vi "PH_PSDBWriter.get PSDB Instance ID.vi"(0 "i ref in":refnum<vi>, 2 "Subsystem":T2 caption="PHELIX Subsysteme" items=["Miscellaneous", "fs-Frontend", "ns-Frontend", "PreAmp", "MainAmp", "MAS", "COS", "Beamline", "Experiment Laserbay", "Experiment Laserlabor", "Experiment Z6", "Timing", "Pulsed Power"], 5 "error in":errorcluster) -> (14 "i ref out":refnum<vi>, 16 "Metadata.Data Status":T1 items=["no info", "no Data collection", "no problem", "Error getting the ID", "Error writing Data", "Error getting the subsystem", "Error getting the Shot ID", "Error getting the Shot Types", "Error getting the Experiments", "Error verifying wanted Shottype", "Error verifying wanted Experiment"], 17 "instance_id":i32, 18 "PSDB Error Code":i32, 19 "error out":errorcluster)   [LabVIEW 2014, in "PH_PSDBWriter.lvlib"]
doc: "This VI get the Instance PHELIX shot data base ID."
uses:
  PH_PSDBWriter.lvlib
  PH_PSDBWriter.PHELIX-Subsystems.ctl
  PH_PSDBWriter.Data Status.ctl
  CSCore/CSSystem/CSSystemLib/CSSystemLib.lvlib
  PH_Common/PH_Common.lvlib
panel:
  in  "PHELIX Subsysteme":T2 items=["Miscellaneous", "fs-Frontend", "ns-Frontend", "PreAmp", "MainAmp", "MAS", "COS", "Beamline", "Experiment Laserbay", "Experiment Laserlabor", "Experiment Z6", "Timing", "Pulsed Power"]
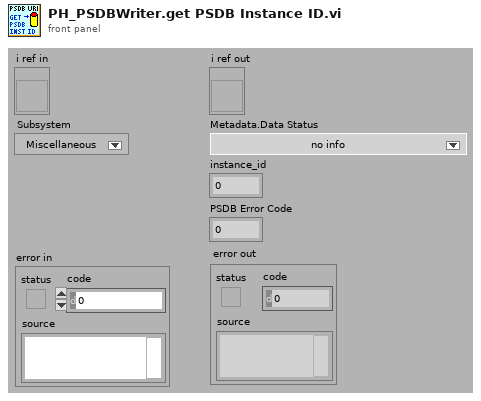
[diagram p1: front panel]
types:
  T1 = typedef "PH_PSDBWriter.lvlib/PH_PSDBWriter.Data Status.ctl" = i16
  T2 = typedef "PH_PSDBWriter.lvlib/PH_PSDBWriter.PHELIX-Subsystems.ctl" = i32
  T3 = typedef "PH_PSDBWriter.lvlib/PH_PSDBWriter.i attribute.ctl" = cluster{"PSDB Status Service ID":i32, "Instance ID":i32, "Shot #":i32, "Subsystem":T2, "Data Status":T1, "Ref PSDB Status":refnum<vi>, "PSDB Error Code":i32, "PSDB Dataset":T4, "PSDB Thread":cluster{"Ref":refnum<vi>, "Q-Ref":refnum<queue>}, "PSDB Credentials":T12}
  T4 = typedef "PH_PSDBWriter.lvlib/PH_PSDBWriter.PSDB Dataset.ctl" = cluster{"Version":i32, "2D data Input":T5[], "Boolean Input":T7[], "Image Input":T8[], "Numeric Input":T10[], "String Input":T11[]}
  T5 = typedef "PH_PSDBWriter.lvlib/PH_PSDBWriter.2D dataset.ctl" = cluster{"name":string, "data":dbl[][], "axis description":T6}
  T6 = typedef "PSDB.lvlib/PSDB_AxisDescription.ctl" = cluster{"x axis label":string, "y axis label":string, "x axis unit":string, "y axis unit":string}
  T7 = typedef "PH_PSDBWriter.lvlib/PH_PSDBWriter.Boolean dataset.ctl" = cluster{"name":string, "data":bool, "unit":string}
  T8 = typedef "PH_PSDBWriter.lvlib/PH_PSDBWriter.Image dataset.ctl" = cluster{"name":string, "data":T9, "unit":string}
  T9 = typedef "IMAQ Image.ctl" = refnum<image>
  T10 = typedef "PH_PSDBWriter.lvlib/PH_PSDBWriter.Numeric dataset.ctl" = cluster{"name":string, "data":dbl, "unit":string}
  T11 = typedef "PH_PSDBWriter.lvlib/PH_PSDBWriter.String dataset.ctl" = cluster{"name":string, "data":string, "unit":string}
  T12 = typedef "PH_Common.lvlib/PH_Connection.PSDB Credentials.ctl" = cluster{"PW":string, "ID":string, "DS":string}
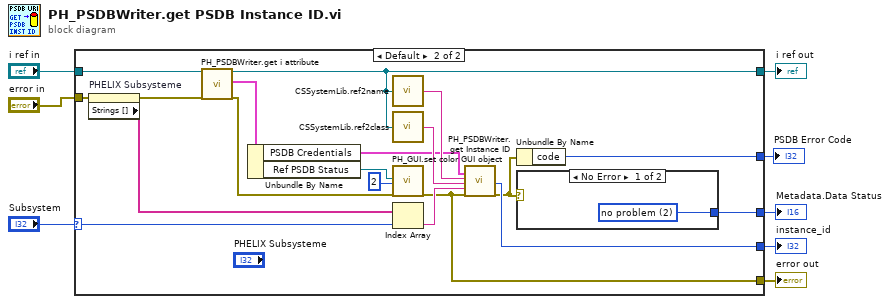
[diagram p0: block diagram]
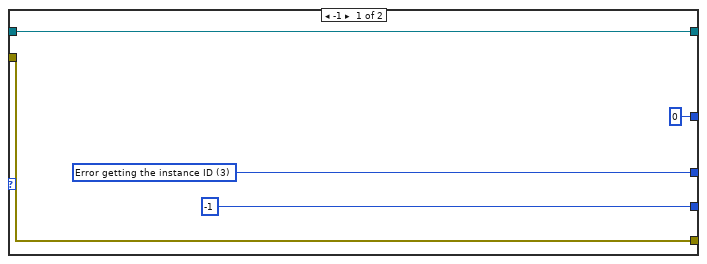
[diagram p2: hidden frame]
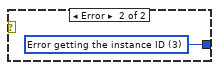
[diagram p3: hidden frame]
diagram:
  n1 = case shown="Default" "Subsystem" {
    selector: "Subsystem" -> [_ w28]
    tunnel: "i ref in" -> [w10 w18]
    tunnel: [w13 w31] -> w7
    tunnel: [-1 ("instance_id") w30] -> w6
    tunnel: "error in" -> [w11 w27]
    tunnel: [w11 w17] -> w3
    tunnel: [w10 w15] -> w2
    tunnel: [0 ("code") w23] -> w1
    frame -1 {
      w13 = T1 3 items=["no info", "no Data collection", "no problem", "Error getting the instance ID", "Error writing Data to data base", "Error concerning the subsystem"] ("Metadata.Data Status")
    }
    frame Default {
      n2 = property on="PHELIX Subsysteme" class="Ring (strict)"(error in=w27) -> (error out=w26:errorcluster, "Strings []"=w29:string[])  [unwired: 1 in, 1 out]
      n3 = call "PH_PSDBWriter.get i attribute.vi"("i ref in"=w18, "error in (no error)"=w26) -> ("i ref out"=w15:refnum<vi>, "i attribute"=w25:T3, "error out"=w21:errorcluster)  [unwired: 15 in]
      n4 = Unbundle By Name(w25) -> ("PSDB Credentials"=w14:T12, "Ref PSDB Status"=w16:refnum<vi>)
      n5 = call "CSSystemLib.ref2name.vi"("obj refnum"=w15) -> ("name"=w20:string)
      n6 = call "CSSystemLib.ref2class.vi"("obj refnum"=w15) -> ("class"=w19:string)
      n7 = call "PH_GUI.set color GUI object.vi"("GUI object Ref"=w16, "State"=2, "error in (no error)"=w21) -> ("error out"=w17:errorcluster)  [unwired: 16 in]
      n8 = Index Array(array=w29, index=w28) -> (element=w32:string)
      n9 = call "PH_PSDBWriter.get Instance ID.vi"("PSDB Credentials"=w14, "Instace Name"=w20, "Class"=w19, "Subsystem"=w32, "error in"=w17) -> ("instance_id"=w30:i32, "error out"=w24:errorcluster)  [unwired: 13 in]
      n10 = Unbundle By Name(w24) -> ("code"=w23:i32)
      n11 = case shown="No Error" w24 {
        tunnel: [w33 w34] -> w31
        frame No Error {
          w33 = T1 2 items=["no info", "no Data collection", "no problem", "Error getting the instance ID", "Error writing Data to data base"] ("Metadata.Data Status")
        }
        frame Error {
          w34 = T1 3 items=["no info", "no Data collection", "no problem", "Error getting the instance ID", "Error writing Data to data base"] ("Metadata.Data Status")
        }
      }
    }
  }
  "Metadata.Data Status" <- w7
  "instance_id" <- w6
  "error out" <- w3
  "i ref out" <- w2
  "PSDB Error Code" <- w1
